vi "ArrayToEnum__A2E.vi"(7 "Control VI Type (control)":T1=enum."control" caption="Control VI Type", 8 "Error In":errorcluster, 9 "Enum Name (Enum)":string caption="Enum Name (FileName)", 10 "Enum Strings":string[](array[string]), 11 "Control Path (use dialog)":path) -> (0 "Error Out":errorcluster)   [LabVIEW 2021, in "Utilities.lvlib"]
doc: "This VI converts an array of strings into an enum with the strings as enum value-strings"
uses:
  Utilities.lvlib
  ControlTypes__A2E.ctl
  Strings/Strings.lvlib
panel:
  out "Duplicate path":path
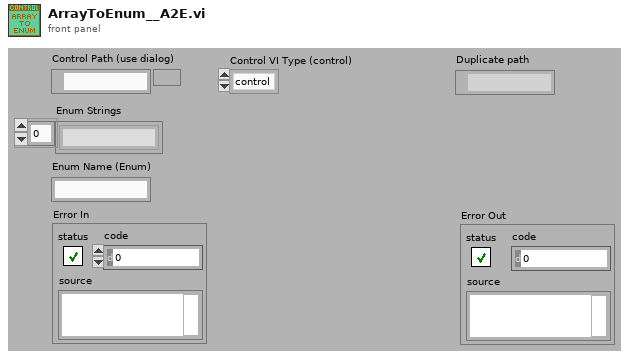
[diagram p1: front panel]
types:
  T1 = typedef "Utilities.lvlib/ControlTypes__A2E.ctl" = enum32{"not a control VI", "control", "typedef", "strict typedef"}
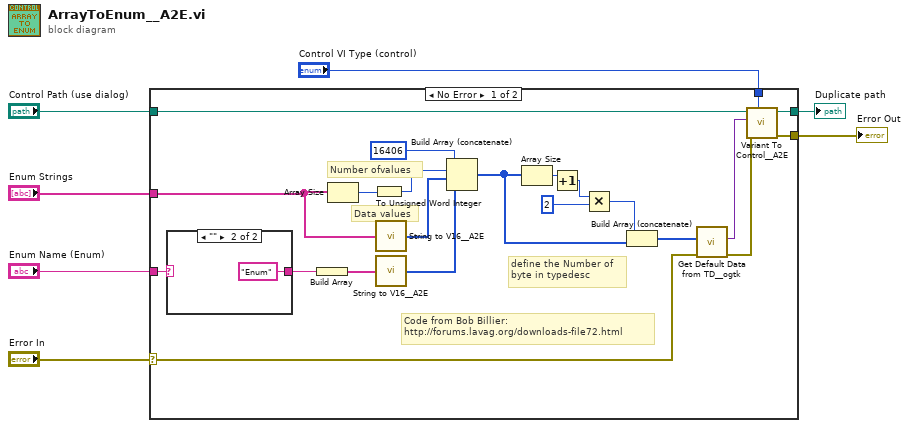
[diagram p0: block diagram]
diagram:
  n1 = case shown="No Error" "Error In" {
    selector: "Error In" -> [w8 w32]
    tunnel: "Enum Strings" -> [w29 _]
    tunnel: "Enum Name (Enum)" -> [w28 _]
    tunnel: [w26 w32] -> w5
    tunnel: "Control VI Type (control)" -> [w15 _]
    tunnel: "Control Path (use dialog)" -> [w10 w33]
    tunnel: [w27 w33] -> w1
    frame No Error {
      # "Code from Bob Billier:\nhttp://forums.lavag.org/downloads-file72.html"
      # "Data values"
      # "Number ofvalues"
      # "define the Number of\nbyte in typedesc"
      n2 = case shown="\"\"" w28 {
        selector: w28 -> [w30 _]
        tunnel: [w30 "Enum"] -> w14
        frame Default {
        }
        frame "" {
        }
      }
      n3 = Build Array(w14) -> (w13:string[])
      n4 = Array Size(array=w29) -> (size(s)=w17:i32)
      n5 = To Unsigned Word Integer(number=w17) -> (unsigned 16bit integer=w16:u16)
      n6 = call "String to V16__A2E.vi"("Array of string Data"=w29) -> ("Array of V16"=w25:u16[])  [unwired: 4 in]
      n7 = call "String to V16__A2E.vi"("Array of string Data"=w13) -> ("Array of V16"=w24:u16[])  [unwired: 4 in]
      n8 = Build Array (concatenate)(u16 16406, w16, w25, w24) -> (w19:u16[])
      n9 = Array Size(array=w19) -> (size(s)=w23:i32)
      n10 = Increment(x=w23) -> (x+1=w22:i32)
      n11 = Multiply(x=w22, y=2) -> (x*y=w20:i32)
      n12 = Build Array (concatenate)(w20, w19) -> (w12:i32[])
      n13 = call <userlib>:"Get Default Data from TD__ogtk.vi"("error in (no error)"=w8, "Type Descriptor"=w12) -> ("error out"=w9:errorcluster, "Default VData"=w11:variant)  [unwired: 8 in]
      n14 = call "Variant To Control__A2E.vi"("Control VI Type (control)"=w15, "Error In"=w9, "Variant Data"=w11, "Control Path (use dialog)"=w10) -> ("error out"=w26:errorcluster, "selected path"=w27:path)  [unwired: 6 in]
    }
    frame Error {
    }
  }
  "Error Out" <- w5
  "Duplicate path" <- w1
